vi "Initialise Objective FOV and AOLZ controls.vi"(8 "error in (no error)":errorcluster, 11 "UI ctrl refs":T1) -> (0 "error out":errorcluster)   [LabVIEW 2017]
uses:
  Typedefs/UI ctrl refs cluster.ctl
  Typedefs/Laser control knob.ctl
  Typedefs/Frame Size.ctl
  Typedefs/Plane Mode.ctl
  Typedefs/PMT control knob.ctl
  User Interface/Misc/Experiment Type.ctl
  User Interface/Misc/Biology Information.ctl
  Global Variables/General Globals.vi
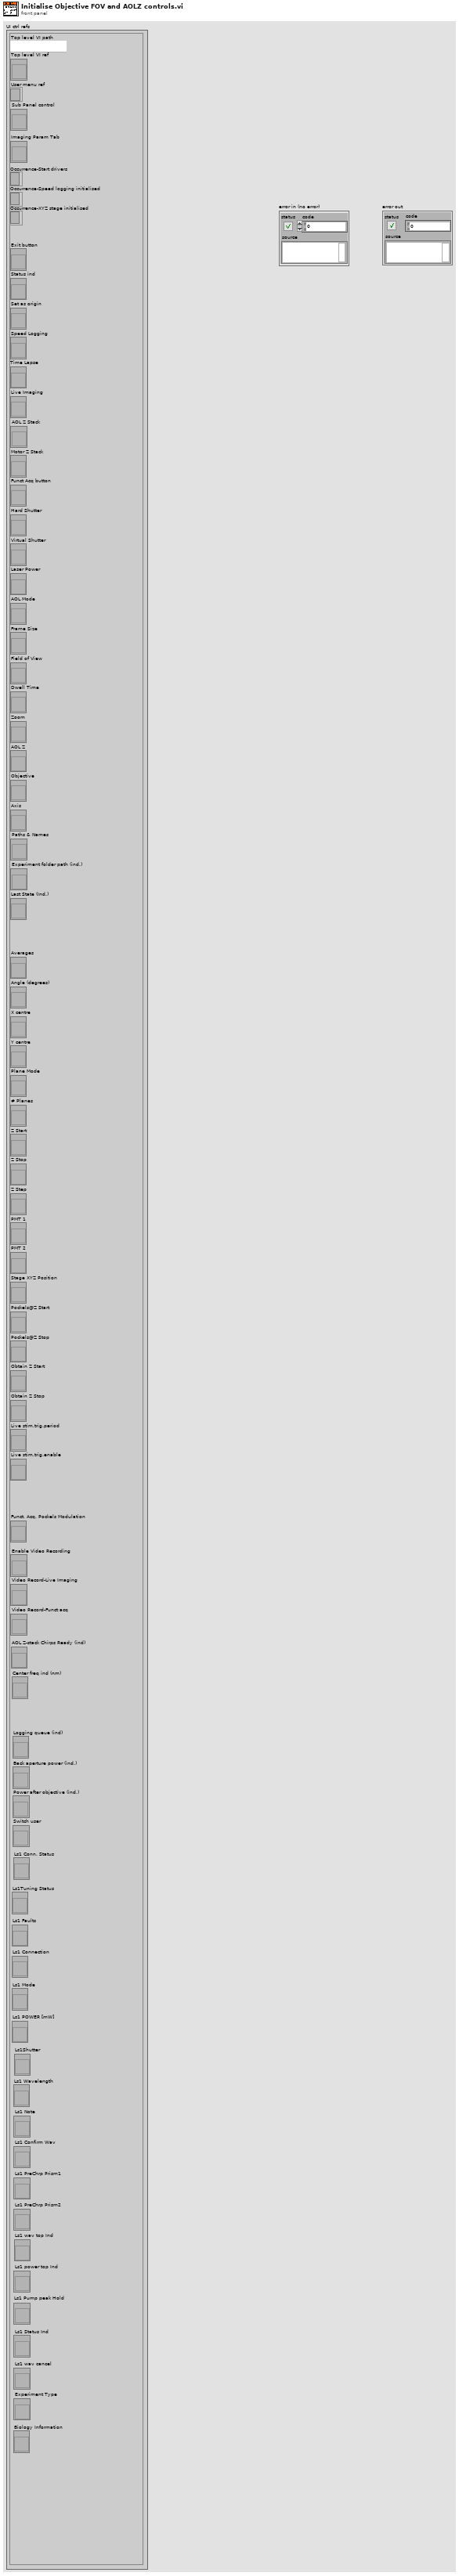
[diagram p1: front panel]
types:
  T1 = typedef "UI ctrl refs cluster.ctl" = cluster{"Top level VI path":path, "Top level VI ref":refnum<vi>, "User menu ref":refnum<k9>, "Sub Panel control":refnum<vi>, "Imaging Param Tab":refnum<vi>, "Occurrence-Start drivers":refnum<k4>, "Occurrence-Speed logging initialised":refnum<k4>, "Occurrence-XYZ stage initialised":refnum<k4>, "Exit button":refnum<vi>, "Status ind":refnum<vi>, "Set as origin":refnum<vi>, "Speed Logging":refnum<vi>, "Time Lapse":refnum<vi>, "Live Imaging":refnum<vi>, "AOL Z Stack":refnum<vi>, "Motor Z Stack":refnum<vi>, "Funct Acq button":refnum<vi>, "Hard Shutter":refnum<vi>, "Virtual Shutter":refnum<vi>, "Laser Power":refnum<vi>, "AOL Mode":refnum<vi>, "Frame Size":refnum<vi>, "Field of View":refnum<vi>, "Dwell Time":refnum<vi>, "Zoom":refnum<vi>, "AOL Z":refnum<vi>, "Objective":refnum<vi>, "Axis":refnum<vi>, "Paths & Names":refnum<vi>, "Experiment folder path (ind.)":refnum<vi>, "Last State (Ind.)":refnum<vi>, "Averages":refnum<vi>, "Angle (degrees)":refnum<vi>, "X centre":refnum<vi>, "Y centre":refnum<vi>, "Plane Mode":refnum<vi>, "# Planes":refnum<vi>, "Z Start":refnum<vi>, "Z Stop":refnum<vi>, "Z Step":refnum<vi>, "PMT 1":refnum<vi>, "PMT 2":refnum<vi>, "Stage XYZ Position":refnum<vi>, "Pockels@Z Start":refnum<vi>, "Pockels@Z Stop":refnum<vi>, "Obtain Z Start":refnum<vi>, "Obtain Z Stop":refnum<vi>, "Live stim.trig.period":refnum<vi>, "Live stim.trig.enable":refnum<vi>, "Funct. Acq. Pockels Modulation":refnum<vi>, "Enable Video Recording":refnum<vi>, "Video Record-Live Imaging":refnum<vi>, "Video Record-Funct acq":refnum<vi>, "AOL Z-stack Chirps Ready (ind)":refnum<vi>, "Center freq ind (nm)":refnum<vi>, "Logging queue (ind)":refnum<vi>, "Back aperture power (ind.)":refnum<vi>, "Power after objective (ind.)":refnum<vi>, "Switch user":refnum<vi>, "Ls1 Conn. Status":refnum<vi>, "Ls1Tuning Status":refnum<vi>, "Ls1 Faults":refnum<vi>, "Ls1 Connection":refnum<vi>, "Ls1 Mode":refnum<vi>, "Ls1 POWER [mW]":refnum<vi>, "Ls1Shutter":refnum<vi>, "Ls1 Wavelength":refnum<vi>, "Ls1 Note":refnum<vi>, "Ls1 Confirm Wav":refnum<vi>, "Ls1 PreChrp Prism1":refnum<vi>, "Ls1 PreChrp Prism2":refnum<vi>, "Ls1 wav top Ind":refnum<vi>, "Ls1 power top Ind":refnum<vi>, "Ls1 Pump peak Hold":refnum<vi>, "Ls1 Status Ind":refnum<vi>, "Ls1 wav cancel":refnum<vi>, "Experiment Type":refnum<vi>, "Biology Information":refnum<vi>}
  T2 = enum16{"Init", "Update Objectives", "Update Current Objective", "Read", "Clear"}
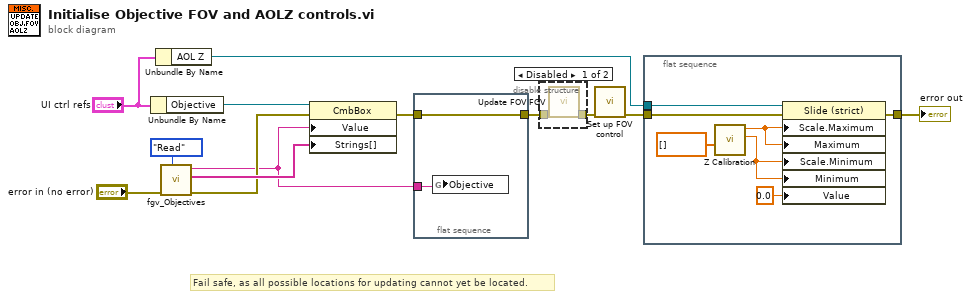
[diagram p0: block diagram]
diagram:
  # "Fail safe, as all possible locations for updating cannot yet be located."
  n1 = Unbundle By Name("UI ctrl refs") -> ("Objective"=w13:refnum<vi>)
  n2 = Unbundle By Name("UI ctrl refs") -> ("AOL Z"=w7:refnum<vi>)
  n3 = call "fgv_Objectives.vi"("Actions"=T2."Read", "error in (no error)"="error in (no error)") -> ("error out"=w9:errorcluster, "Objectives"=w11:string[], "Current Objective"=w1:string)  [unwired: 7 in]
  n4 = property class="CmbBox"(reference=w13, error in=w9, "Value"=w1, "Strings[]"=w11) -> (error out=w3:errorcluster)  [unwired: 1 out]
  n5 = flat-sequence {
    tunnel: w1 -> [w15]
    tunnel: w3 -> [w14]
    tunnel: [w14] -> w2
    frame #0 {
      n6 = global write "General Globals.vi" "Objective"(w15) -> ()
    }
  }
  n7 = disable-structure shown="Disabled" {
    disable-tunnel: [w17 w18] -> w8
    disable-tunnel: w2 -> [w16 w18]
    frame Disabled {
      n8 = call "Update FOV FGV.vi"("error in (no error)"=w16) -> ("error out"=w17:errorcluster)  [unwired: 10 in]
    }
    frame Enabled {
    }
  }
  n9 = call "Set up FOV control.vi"("error in (no error)"=w8) -> ("error out"=w5:errorcluster)  [unwired: 10 in]
  n10 = flat-sequence {
    tunnel: w7 -> [w24]
    tunnel: w5 -> [w20]
    tunnel: [w19] -> w4
    frame #0 {
      n11 = call "Z Calibration.vi"("Z Planes"=dbl[] [] ("Motor Z")) -> ("Z Min"=w22:dbl, "Z Max"=w23:dbl)  [unwired: 7 in, 2 out]
      n12 = property on="Property Node" class="Slide (strict)"(reference=w24, error in=w20, "Scale.Maximum"=w23, "Maximum"=w23, "Scale.Minimum"=w22, "Minimum"=w22, "Value"=sgl 0.0) -> (error out=w19:errorcluster)  [unwired: 1 out]
    }
  }
  "error out" <- w4
